vi "Speed Control 1 - Halfway through.vi"(11 "queue in":refnum<queue>) -> ()   [LabVIEW 2014]
uses:
  controls/UI Data.ctl
  controls/Control ConfigurationSam.ctl
  controls/EncoderController.ctl
  <vilib>/Platform/TimedLoop/XDataNode/timing_clust.ctl
  <vilib>/Platform/TimedLoop/XDataNode/nitl_modes.ctl
  <vilib>/Platform/TimedLoop/XDataNode/wakeup.ctl
  controls/Control StateSam.ctl
  <vilib>/Platform/TimedLoop/XDataNode/loadnilvce.vi
  <vilib>/addons/control/pid/pid.llb/PID (DBL).vi
  <vilib>/addons/control/pid/pid.llb/PID Percentage to EGU (DBL).vi
  <vilib>/platform/TimedLoop/XDataNode/XDataNode.xnode
  <vilib>/addons/control/pid/NI_PID_pid.lvlib
  <vilib>/Platform/TimedLoop/XDataNode/XDNodeRunTimeDep.lvlib
panel:
  out "Velocity4 RPM":dbl
  out "Ch 4 Setpoint":dbl
  out "Motor1Output":dbl
  out "Velocity1 RPM":dbl
  # "0.8, 0. 0 is stable but theres a large offset\nsystem is slow to settle, increase Ti"
  # "Kp=2.04, Ti=0.15, Td=0.0375"
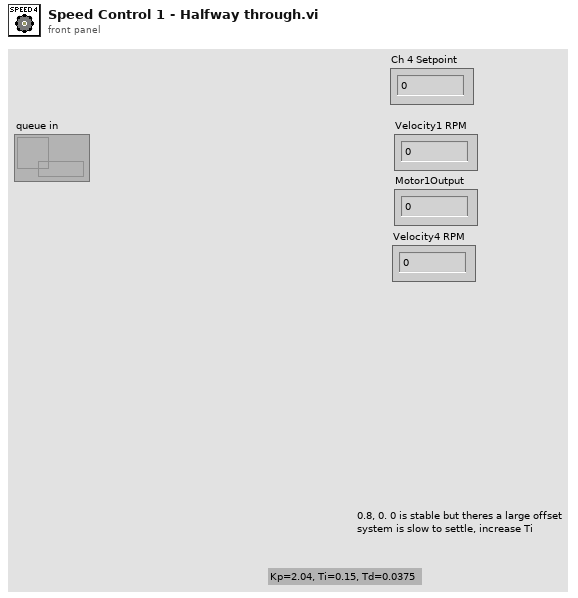
[diagram p1: front panel]
types:
  T1 = typedef "Control ConfigurationSam.ctl" = cluster{"PID Gains":cluster{"proportional gain (Kc)":dbl, "integral gain (Kc*Ts/Ti)":dbl, "derivative gain (Kc*Td/Ts)":dbl}, "Output Range":cluster{"output high":dbl, "output low":dbl}}
  T2 = cluster{bool, "Tick Count(uSec)":u32, "Counter Value":i32, "x-y":i32}
  T3 = cluster{"proportional gain (Kc)":dbl, "integral gain (Kc*Ts/Ti)":dbl, "derivative gain (Kc*Td/Ts)":dbl}
  T4 = cluster{"proportional gain (Kc)":dbl, "integral gain (Kc*Ts/Ti)":dbl, "derivative gain (Kc*Td/Ts)":dbl}[]
  T5 = typedef "XDNodeRunTimeDep.lvlib/timing_clust.ctl" = cluster{"Expected End [f-1]":u64, "Actual End [f-1]":u64, "Finished Late? [f-1]":bool, "Expected End [i-1]":u64, "Actual End [i-1]":u64, "Finished Late? [i-1]":bool, "Expected Start [i]":u64, "Actual Start [i]":u64, "Expected Start [f]":u64, "Actual Start [f]":u64, "Source Name":string, "Structure Name":string, "Period":i64, "Deadline":i64, "Offset":i64, "Start":i64, "Priority":i32, "Timeout":i32, "Mode":T6, "Wakeup Reason":T7, "Error":errorcluster, "Source Type":string, "Secondary Source Type":string, "Global End Time":u64, "Global Start Time":u64, "Frame Duration":u64, "Iteration Duration":u64, "Assigned CPU":i32, "I/O Scan Engine Mode":u32}
  T6 = typedef "XDNodeRunTimeDep.lvlib/nitl_modes.ctl" = enum32{"No Change", "Process missed periods, maintain original phase", "Discard missed periods, maintain original phase", "Process missed periods, ignore original phase", "Discard missed periods, ignore original phase"}
  T7 = typedef "XDNodeRunTimeDep.lvlib/wakeup.ctl" = enum32{"Normal", "Aborted", "Asynchronous wakeup", "Timing source error", "Timed loop error", "Timeout"}
  T8 = typedef "Control StateSam.ctl" = enum16{"", "Control State (PID)", "Safe State"}
  T9 = typedef "EncoderController.ctl" = cluster{"Sample time (uS)":u32, "Reset":bool}
  T10 = typedef "EncoderIndicator.ctl" = cluster{"Position":dbl, "Velocity RPM":dbl, "Velocity RPS":dbl}
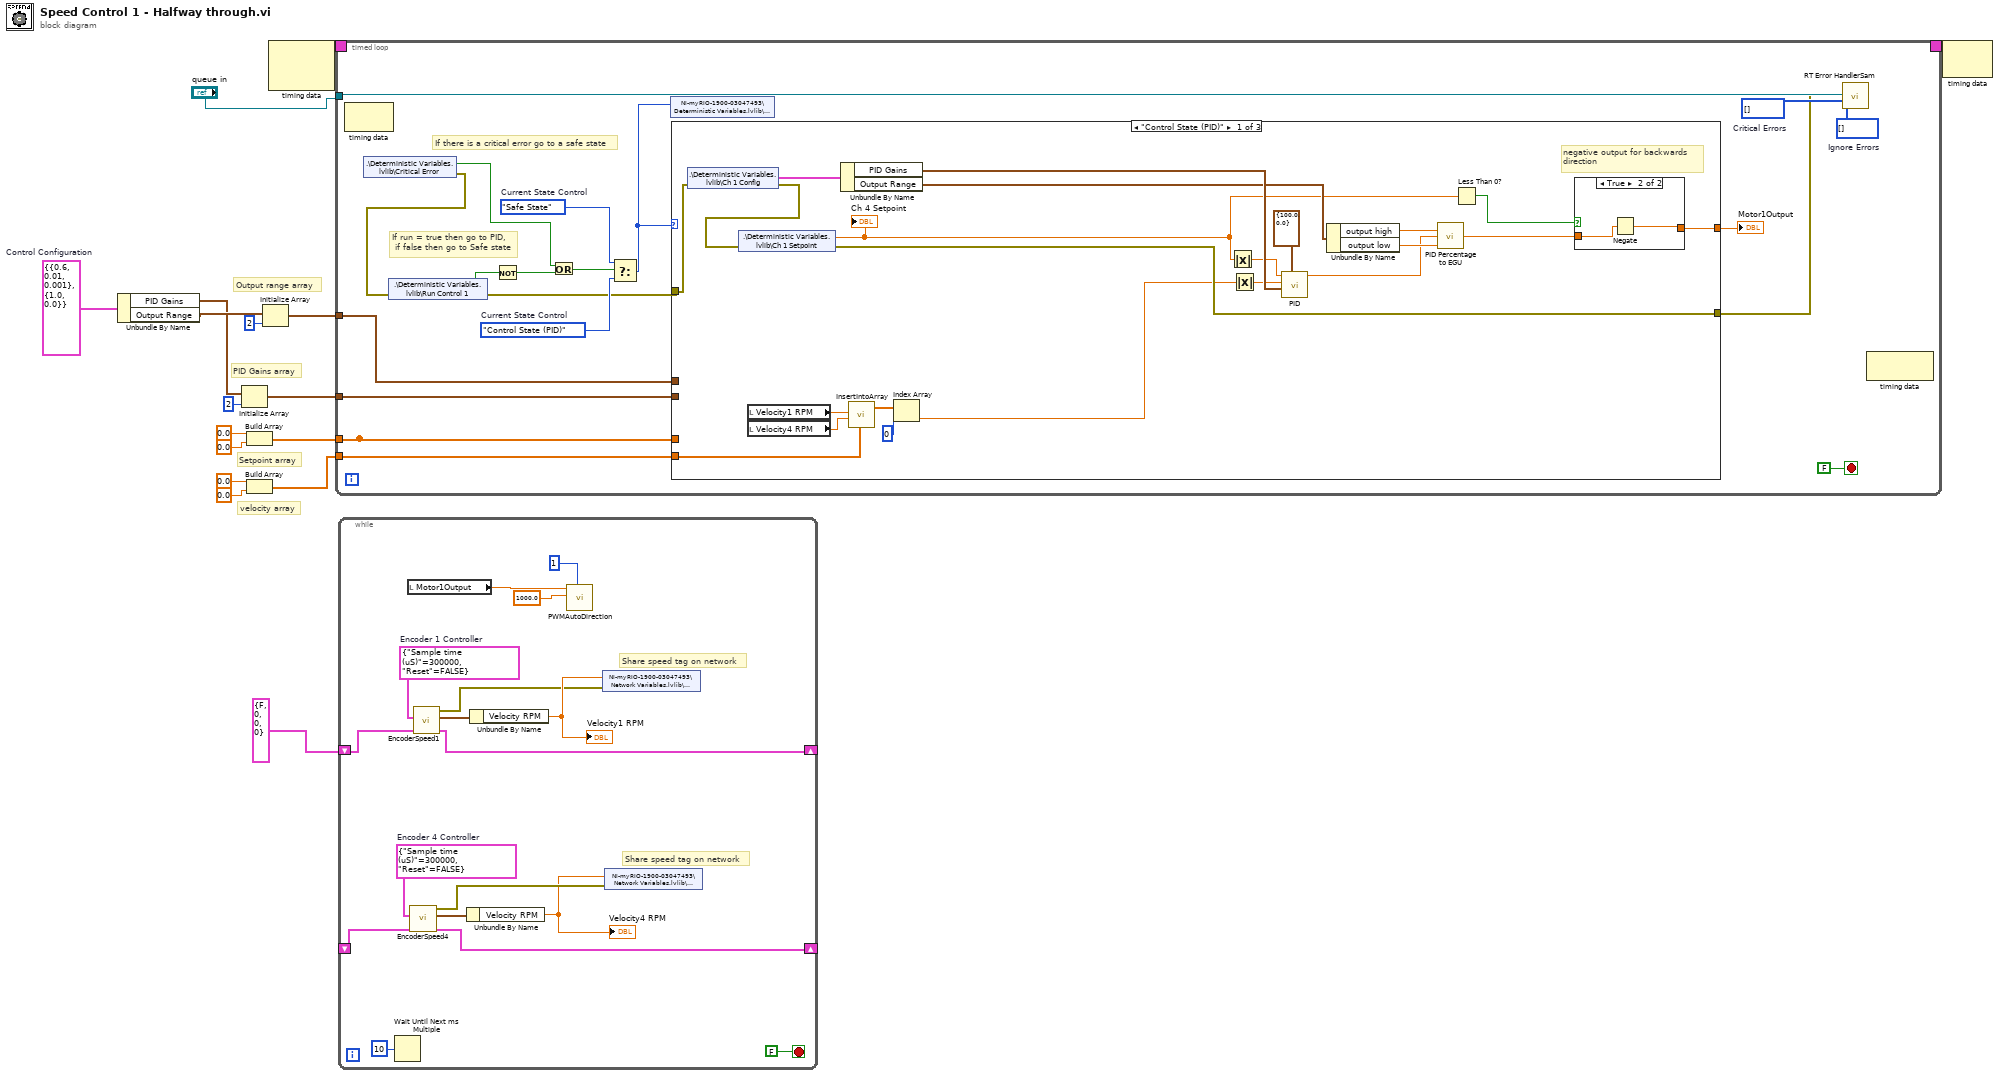
[diagram p0: block diagram]
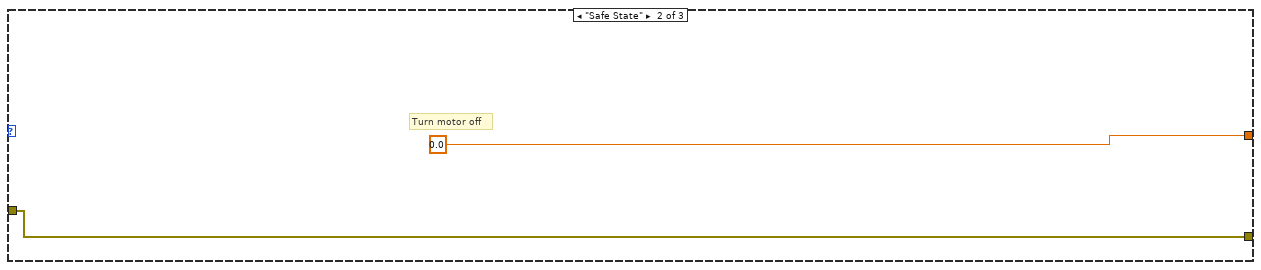
[diagram p3: hidden frame]
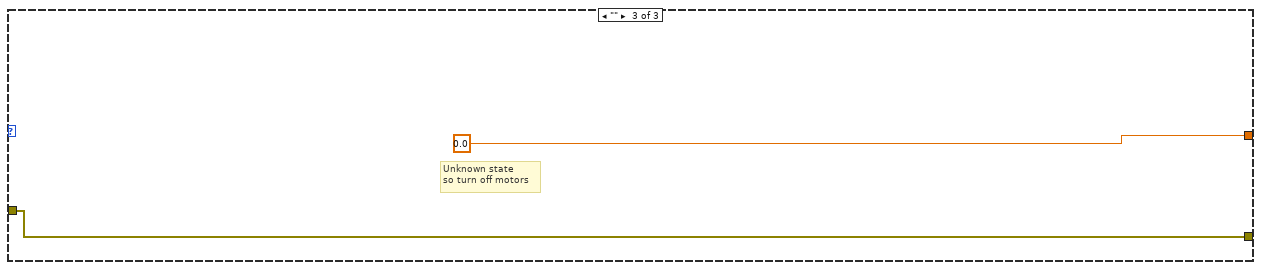
[diagram p4: hidden frame]
diagram:
  w10 = T1 {"PID Gains"={"proportional gain (Kc)"=0.6, "integral gain (Kc*Ts/Ti)"=0.01, "derivative gain (Kc*Td/Ts)"=0.001}, "Output Range"={"output high"=1.0, "output low"=0.0}}  # Control Configuration
  # "Output range array"
  # "velocity array"
  # "PID Gains array"
  # "Setpoint array"
  n1 = Unbundle By Name(w10) -> ("PID Gains"=w11:T3, "Output Range"=w13:cluster{"output high":dbl, "output low":dbl})
  n2 = Initialize Array(w11, 2 ("dimension size")) -> (w3:T4)
  n3 = Build Array(0.0, 0.0) -> (w2:dbl[])
  n4 = Build Array(0.0, 0.0) -> (w1:dbl[])
  n5 = Initialize Array(w13, 2 ("dimension size")) -> (w4:cluster{"output high":dbl, "output low":dbl}[])
  n6 = node-c288() -> (w17:T5)  [unwired: 2 in]
  n7 = timed-loop {
    timing: w17 -> [_]
    timing-out: [_] -> w16
    tunnel: "queue in" -> [w24]
    tunnel: w4 -> [w18]
    tunnel: w3 -> [w19]
    tunnel: [w20] -> _
    tunnel: w2 -> [w20]
    tunnel: w1 -> [w21]
    stop <- FALSE stop-if-true
    w25 = i32[] []  # Critical Errors
    w26 = i32[] []  # Ignore Errors
    w33 = Control_StateSam."Control State (PID)"  # Current State Control
    w34 = Control_StateSam."Safe State"  # Current State Control
    # "If there is a critical error go to a safe state"
    # "If run = true then go to PID,\n if false then go to Safe state"
    n8 = node-c288() -> ()  [unwired: 1 in, 1 out]
    n9 = shared-variable ".\\Deterministic Variables.lvlib\\Critical Error"() -> (w30:bool, error out=w28:errorcluster)  [unwired: 1 in]
    n10 = shared-variable ".\\Deterministic Variables.lvlib\\Run Control 1"(error in=w28) -> (w35:bool, error out=w27:errorcluster)
    n11 = Not(x=w35) -> (.not. x?=w31:bool)
    n12 = Or(x=w30, y=w31) -> (x .or. y?=w29:bool)
    n13 = Select(t=w34, s=w29, f=w33) -> (s? t:f=w32:T8)
    n14 = shared-variable "NI-myRIO-1900-03047493\\Deterministic Variables.lvlib\\Control State 1"(w32) -> ()  [unwired: 1 in, 1 out]
    n15 = case shown="\"Control State (PID)\"" w32 {
      tunnel: [w46 0.0 ("output (EGU)") 0.0 ("output (EGU)")] -> w23
      tunnel: w27 -> [w51 w62 w64]
      tunnel: [w49 w62 w64] -> w22
      tunnel: w21 -> [w40 _ _]
      tunnel: w20 -> [_ _ _]
      tunnel: w19 -> [_ _ _]
      tunnel: w18 -> [_ _ _]
      frame "Control State (PID)" {
        # "negative output for backwards \ndirection"
        n16 = shared-variable ".\\Deterministic Variables.lvlib\\Ch 1 Config"(error in=w51) -> (w55:T1, error out=w50:errorcluster)
        n17 = shared-variable ".\\Deterministic Variables.lvlib\\Ch 1 Setpoint"(error in=w50) -> (w45:dbl, error out=w49:errorcluster)
        "Ch 4 Setpoint" <- w45
        n18 = local read "Velocity1 RPM"() -> (w42:dbl)
        n19 = local read "Velocity4 RPM"() -> (w41:dbl)
        n20 = Unbundle By Name(w55) -> ("PID Gains"=w56:T3, "Output Range"=w53:cluster{"output high":dbl, "output low":dbl})
        n21 = call "InsertIntoArray.vi"("input array"=w40, "new element 1"=w41, "new element 0"=w42) -> ("output array"=w39:dbl[])  [unwired: 8 in]
        n22 = Index Array(array=w39, index=0) -> (element=w37:dbl)
        n23 = Absolute Value(x=w45) -> (abs(x)=w44:dbl)
        n24 = Absolute Value(x=w37) -> (abs(x)=w43:dbl)
        n25 = call-poly <vilib>:"PID.vi"("output range"=cluster{"output high":dbl, "output low":dbl} {"output high"=100.0, "output low"=0.0}, "PID gains"=w56, "process variable"=w43, "setpoint"=w44) -> ("output"=w54:dbl)  [unwired: 6 in, 1 out]
        n26 = Unbundle By Name(w53) -> ("output high"=w58:dbl, "output low"=w57:dbl)
        n27 = call-poly <vilib>:"PID Percentage to EGU.vi"("minimum (EGU)"=w57, "% span"=w54, "maximum (EGU)"=w58) -> ("output (EGU)"=w47:dbl)  [unwired: 1 in]
        n28 = Less Than 0?(x=w45) -> (x < 0?=w48:bool)
        n29 = case shown="True" w48 {
          tunnel: w47 -> [w59 w61]
          tunnel: [w59 w60] -> w46
          frame False {
          }
          frame True {
            n30 = Negate(x=w61) -> (-x=w60:dbl)
          }
        }
      }
      frame "Safe State" {
        # "Turn motor off"
      }
      frame "" {
        # "Unknown state\nso turn off motors"
      }
    }
    "Motor1Output" <- w23
    n31 = call "RT Error HandlerSam.vi"("Ignore Errors"=w26, "Critical Errors"=w25, "error to process"=w22, "queue in"=w24) -> ()  [unwired: 7 in, 1 out]
    n32 = node-c288() -> ()  [unwired: 1 in, 1 out]
  }
  n33 = while {
    shift-right: [w79] -> _
    shift-left: T2 {FALSE, "Tick Count(uSec)"=0, "Counter Value"=0, "x-y"=0} ("Cluster out") -> [w80]
    shift-right: [w69] -> _
    shift-left: _ -> [w70]
    stop <- FALSE stop-if-true
    w71 = T9 {"Sample time (uS)"=300000, "Reset"=FALSE}  # Encoder 4 Controller
    w84 = T9 {"Sample time (uS)"=300000, "Reset"=FALSE}  # Encoder 1 Controller
    # "Share speed tag on network"
    # "Share speed tag on network"
    n34 = Wait Until Next ms Multiple(millisecond multiple=u32 10) -> ()  [unwired: 1 out]
    n35 = local read "Motor1Output"() -> (w76:dbl)
    n36 = call "EncoderSpeed4.vi"("Cluster in"=w70, "Encoder 4 Controller"=w71) -> ("Cluster out"=w69:T2, "Encoder 4 Indicator"=w72:T10, "error out"=w73:errorcluster)  [unwired: 7 in]
    n37 = call "EncoderSpeed1.vi"("Cluster in"=w80, "Encoder 1 Controller"=w84) -> ("Cluster out"=w79:T2, "Encoder 1 Indicator"=w83:T10, "error out"=w81:errorcluster)  [unwired: 7 in]
    n38 = Unbundle By Name(w72) -> ("Velocity RPM"=w68:dbl)
    "Velocity4 RPM" <- w68
    n39 = Unbundle By Name(w83) -> ("Velocity RPM"=w82:dbl)
    "Velocity1 RPM" <- w82
    n40 = call "PWMAutoDirection.vi"("Motor Select"=i8 1, "PWM Frequency"=1000.0, "DutyCycle"=w76) -> ()  [unwired: 8 in, 1 out]
    n41 = shared-variable "NI-myRIO-1900-03047493\\Network Variables.lvlib\\SpeedMotor1"(w82, error in=w81) -> ()  [unwired: 1 out]
    n42 = shared-variable "NI-myRIO-1900-03047493\\Network Variables.lvlib\\SpeedMotor4"(w68, error in=w73) -> ()  [unwired: 1 out]
  }
  n43 = node-c288(w16) -> ()  [unwired: 1 out]
